vi "COMLOGQueue-Write.vi"(5 "COM(Constant)":string, 8 "element":string, 9 "Prefix":string) -> (3 "queue":refnum<queue>)   [LabVIEW 2020]
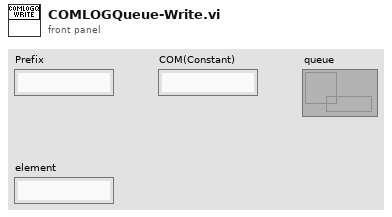
[diagram p1: front panel]
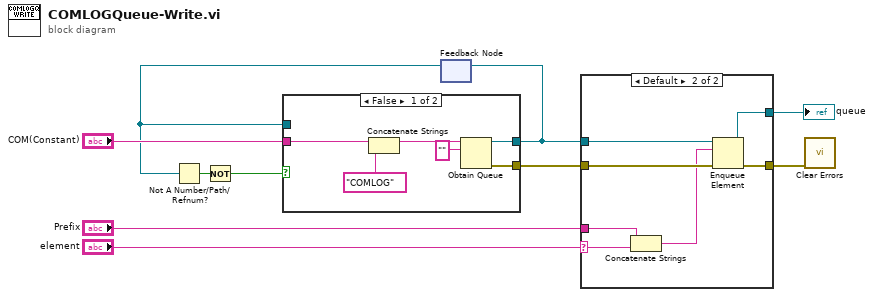
[diagram p0: block diagram]
diagram:
  n1 = feedback #1() -> (w8:refnum<queue>)  [unwired: 1 in]
  n2 = Not A Number/Path/Refnum?(number/path/refnum=w8) -> (NaN/Path/Refnum?=w1:bool)
  n3 = Not(x=w1) -> (.not. x?=w9:bool)
  n4 = case shown="False" w9 {
    tunnel: "COM(Constant)" -> [w16 _]
    tunnel: [w14 w17] -> w7
    tunnel: w8 -> [_ w17]
    tunnel: [w11 _] -> w6
    frame False {
      n5 = Concatenate Strings(w16, "COMLOG" ("string")) -> (w13:string)
      n6 = Obtain Queue(name (unnamed)=w13, element data type="") -> (queue out=w14:refnum<queue>, error out=w11:errorcluster)  [unwired: 3 in, 1 out]
    }
    frame True {
    }
  }
  n7 = feedback-in #1(w7) -> ()
  n8 = case shown="Default" "element" {
    selector: "element" -> [_ w20]
    tunnel: w7 -> [w19 w26]
    tunnel: w6 -> [w18 w25]
    tunnel: [w18 w24] -> w5
    tunnel: [w19 w23] -> w4
    tunnel: "Prefix" -> [_ w22]
    frame "" {
    }
    frame Default {
      n9 = Concatenate Strings(w22, w20) -> (w21:string)
      n10 = Enqueue Element(queue=w26, element=w21, error in (no error)=w25) -> (queue out=w23:refnum<queue>, error out=w24:errorcluster)  [unwired: 1 in, 1 out]
    }
  }
  "queue" <- w4
  n11 = call <vilib>:"Clear Errors.vi"("error in (no error)"=w5) -> ()  [unwired: 5 in, 2 out]
